vi "getPropertySelectionValue.vi"(8 "error in (no error)":errorcluster, 10 "Property Name in":string, 11 "IPropertyObject in":refnum<class "IPropertyObject.lvclass">) -> (0 "error out":errorcluster, 1 "Property Selection Value out":refnum<class "IBaseObject.lvclass">, 2 "Property Name out":string, 3 "IPropertyObject out":refnum<class "IPropertyObject.lvclass">)   [LabVIEW 2022 SP3, in "openDAQ.lvlib" / "IBaseObject.lvlib" / "IPropertyObject.lvlib" / "IPropertyObject.lvclass"]
uses:
  <instrlib>/openDAQ/Public/Classes/IPropertyObject/IPropertyObject.lvclass
  C:/Program Files (x86)/National Instruments/LabVIEW 2022/instr.lib/openDAQ/Public/Classes/IBaseObject/IBaseObject.lvclass
  <instrlib>/openDAQ/Public/Classes/IBaseObject/IBaseObject.lvclass
  <instrlib>/openDAQ/Public/Classes/IBaseObject/IBaseObject.lvclass/IBaseObject.ctl
  <instrlib>/openDAQ/Public/Classes/IBaseObject/Accessor/Read reference.vi
  <instrlib>/openDAQ/Public/Classes/IBaseObject/Accessor/Write reference.vi
  <instrlib>/openDAQ/Public/Classes/daqCoreTypes/IString/IString.lvclass
  <instrlib>/openDAQ/Binaries/Windows/x86/copendaq32.dll
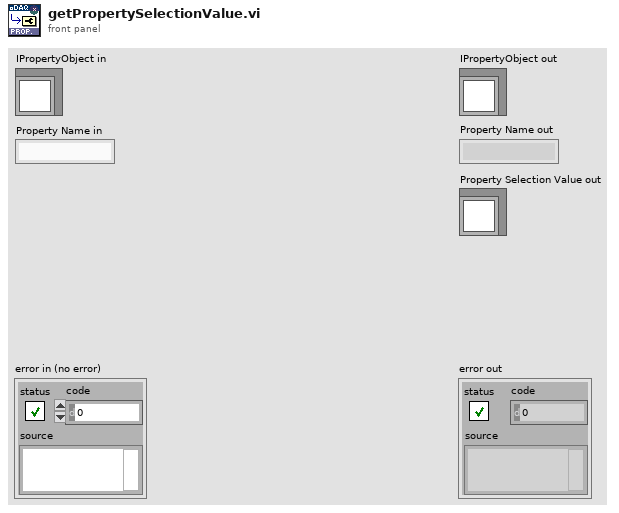
[diagram p1: front panel]
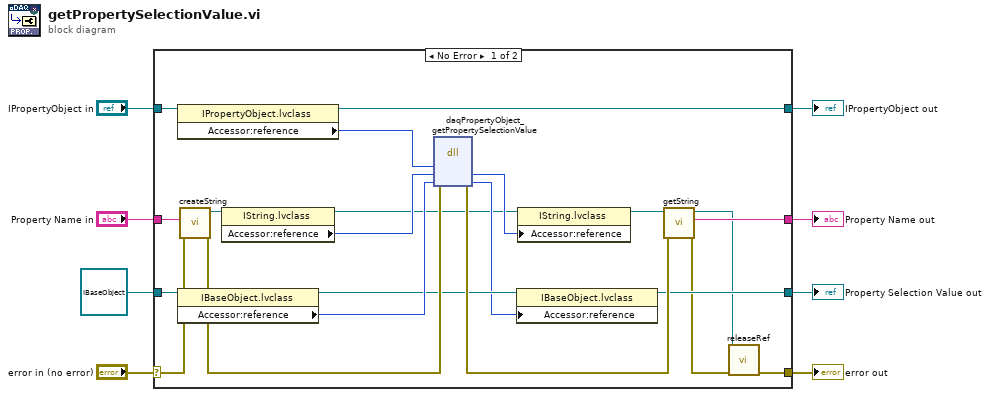
[diagram p0: block diagram]
diagram:
  n1 = case shown="No Error" "error in (no error)" {
    selector: "error in (no error)" -> [w24 w33]
    tunnel: [w13 w33] -> w7
    tunnel: [w25 w32] -> w5
    tunnel: "IPropertyObject in" -> [w27 w32]
    tunnel: "Property Name in" -> [w22 w30]
    tunnel: refnum<class "IBaseObject.lvclass"> refnum ("openDAQ.lvlib:IBaseObject.lvlib:IBaseObject.lvclass") -> [w21 w31]
    tunnel: [w18 w31] -> w1
    tunnel: [w15 w30] -> w2
    frame No Error {
      n2 = property class="IPropertyObject.lvclass"(reference=w27) -> (reference out=w25:refnum<class "IPropertyObject.lvclass">, "Accessor:reference"=w26:i64)  [unwired: 1 in, 1 out]
      n3 = property class="IBaseObject.lvclass"(reference=w21) -> (reference out=w19:refnum<class "IBaseObject.lvclass">, "Accessor:reference"=w29:i64)  [unwired: 1 in, 1 out]
      n4 = call <instrlib>:"createString.vi"("error in (no error)"=w24, "String"=w22) -> ("error out"=w23:errorcluster, "IString out"=w20:refnum<class "IString.lvclass">)  [unwired: 8 in]
      n5 = property class="IString.lvclass"(reference=w20) -> (reference out=w9:refnum<class "IString.lvclass">, "Accessor:reference"=w17:i64)  [unwired: 1 in, 1 out]
      n6 = dll-call lib="C:/Program Files (x86)/National Instruments/LabVIEW 2022/instr.lib/openDAQ/Binaries/Windows/x86/copendaq*.*" fn="daqPropertyObject_getPropertySelectionValue"(error in=w23, "propertyObject"=w26, "name"=w17, "selectionValue"=w29) -> (error out=w28:errorcluster, "name"=w11:i64, "selectionValue"=w10:i64)  [unwired: 4 in, 1 out]
      n7 = property class="IBaseObject.lvclass"(reference=w19, "Accessor:reference"=w10) -> (reference out=w18:refnum<class "IBaseObject.lvclass">)  [unwired: 1 in, 1 out]
      n8 = property class="IString.lvclass"(reference=w9, "Accessor:reference"=w11) -> (reference out=w16:refnum<class "IString.lvclass">)  [unwired: 1 in, 1 out]
      n9 = call <instrlib>:"getString.vi"("error in (no error)"=w28, "IString in"=w16) -> ("error out"=w14:errorcluster, "String out"=w15:string, "IString out"=w12:refnum<class "IString.lvclass">)  [unwired: 7 in]
      n10 = call-dynamic "releaseRef.vi"("error in (no error)"=w14, "IBaseObject in"=w12) -> ("error out"=w13:errorcluster)  [unwired: 9 in]
    }
    frame Error {
    }
  }
  "error out" <- w7
  "IPropertyObject out" <- w5
  "Property Name out" <- w2
  "Property Selection Value out" <- w1
